vi "Average RGB Colors.vi"(9 "Transparency Factor":dbl, 10 "x":u32(colorbox), 11 "y":u32(colorbox)) -> (3 "result":u32(colorbox))   [LabVIEW 2012, in "Picture Box Tools.lvlib"]
uses:
  Picture Box Tools.lvlib
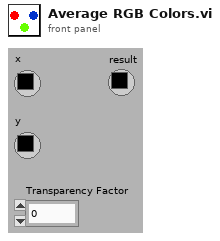
[diagram p1: front panel]
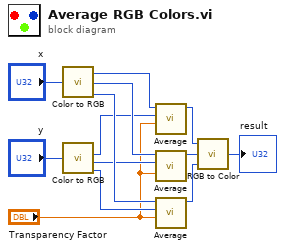
[diagram p0: block diagram]
diagram:
  n1 = call <vilib>:"Color to RGB.vi"("Color"="x") -> ("R"=w7:u8, "G"=w6:u8, "B"=w5:u8)  [unwired: 1 out]
  n2 = call <vilib>:"Color to RGB.vi"("Color"="y") -> ("R"=w2:u8, "G"=w3:u8, "B"=w4:u8)  [unwired: 1 out]
  n3 = call "Average.vi"("Transparency Factor"="Transparency Factor", "x"=w2, "y"=w7) -> ("z"=w10:u8)  [unwired: 8 in]
  n4 = call "Average.vi"("Transparency Factor"="Transparency Factor", "x"=w3, "y"=w6) -> ("z"=w9:u8)  [unwired: 8 in]
  n5 = call "Average.vi"("Transparency Factor"="Transparency Factor", "x"=w4, "y"=w5) -> ("z"=w8:u8)  [unwired: 8 in]
  n6 = call <vilib>:"RGB to Color.vi"("B"=w8, "G"=w9, "R"=w10) -> ("Color"=→"result":u32)
